vi "HodieWindow.vi"(5 "Input":waveform(dbl)(graph)) -> (2 "Output":waveform(dbl)(graph))   [LabVIEW 2019]
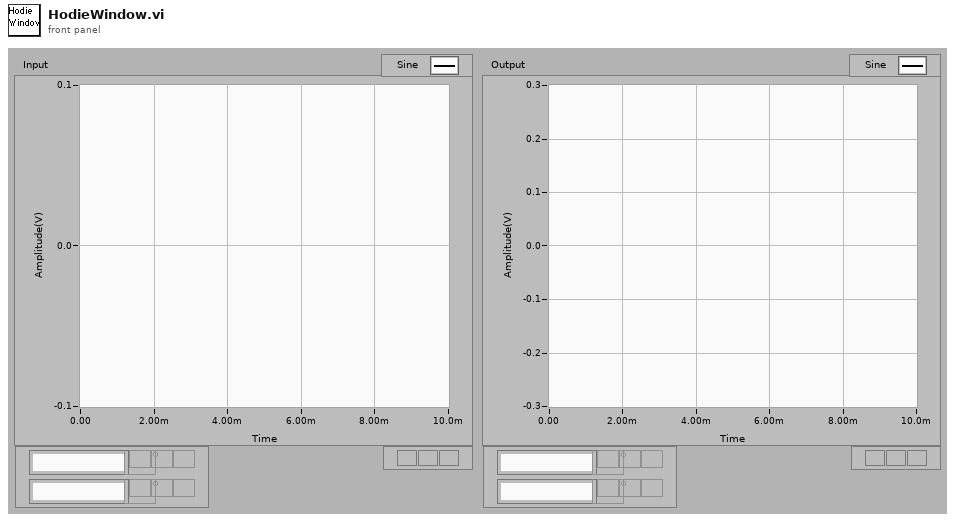
[diagram p1: front panel]
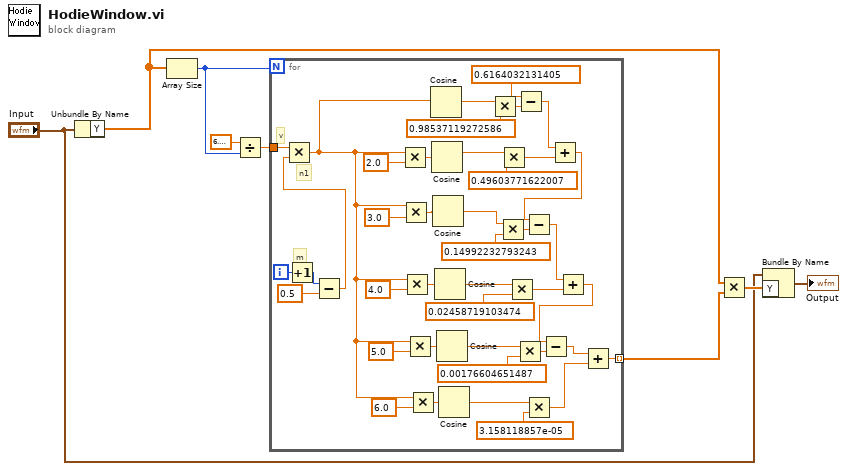
[diagram p0: block diagram]
diagram:
  n1 = Unbundle By Name("Input") -> ("Y"=w5:dbl[])
  n2 = Array Size(array=w5) -> (size(s)=w1:i32)
  n3 = Divide(x=6.283185307179586, y=w1) -> (x/y=w7:dbl)
  n4 = for {
    N: w1 -> [_]
    tunnel: w7 -> [w23]
    tunnel: [w26] -> w6 mode=indexing
    i -> [w22]
    # "n1"
    # "m"
    # "v"
    n5 = Increment(x=w22) -> (x+1=w9:i32)
    n6 = Subtract(x=w9, y=0.5) -> (x-y=w21:dbl)
    n7 = Multiply(x=w23, y=w21) -> (x*y=w15:dbl)
    n8 = Multiply(x=w15, y=2.0) -> (x*y=w20:dbl)
    n9 = Multiply(x=w15, y=3.0) -> (x*y=w19:dbl)
    n10 = Multiply(x=w15, y=4.0) -> (x*y=w18:dbl)
    n11 = Multiply(x=w15, y=5.0) -> (x*y=w17:dbl)
    n12 = Multiply(x=w15, y=6.0) -> (x*y=w16:dbl)
    n13 = Cosine(x=w15) -> (cos(x)=w45:dbl)
    n14 = Cosine(x=w20) -> (cos(x)=w42:dbl)
    n15 = Cosine(x=w19) -> (cos(x)=w35:dbl)
    n16 = Cosine(x=w18) -> (cos(x)=w33:dbl)
    n17 = Cosine(x=w17) -> (cos(x)=w24:dbl)
    n18 = Cosine(x=w16) -> (cos(x)=w25:dbl)
    n19 = Multiply(x=w45, y=0.98537119272586) -> (x*y=w46:dbl)
    n20 = Multiply(x=w35, y=0.14992232793243) -> (x*y=w38:dbl)
    n21 = Multiply(x=w42, y=0.49603771622007) -> (x*y=w47:dbl)
    n22 = Multiply(x=w33, y=0.02458719103474) -> (x*y=w37:dbl)
    n23 = Multiply(x=w24, y=0.00176604651487) -> (x*y=w30:dbl)
    n24 = Subtract(x=0.6164032131405, y=w46) -> (x-y=w43:dbl)
    n25 = Multiply(x=w25, y=3.158118857e-05) -> (x*y=w31:dbl)
    n26 = Add(x=w43, y=w47) -> (x+y=w34:dbl)
    n27 = Subtract(x=w34, y=w38) -> (x-y=w39:dbl)
    n28 = Add(x=w39, y=w37) -> (x+y=w27:dbl)
    n29 = Subtract(x=w27, y=w30) -> (x-y=w29:dbl)
    n30 = Add(x=w29, y=w31) -> (x+y=w26:dbl)
  }
  n31 = Multiply(x=w5, y=w6) -> (x*y=w4:dbl[])
  n32 = Bundle By Name(cluster="Input", "Y"=w4) -> (→"Output":waveform(dbl))
